vi "CMD_Codec.vi"() -> ()   [LabVIEW 2025]
uses:
  <vilib>/addons/JSON API/JSON Value/Set from JSON string.vi
  <vilib>/addons/JSON API/JSON Value/JSON Value.lvclass
  <vilib>/addons/JSON API/JSON Value/Get sub-Item by names.vi
  <vilib>/addons/JSON API/JSON Scalar/Get as Text.vi
  <vilib>/addons/JSON API/Get Polymorphic/JSON GetSet.lvlib
  <vilib>/addons/JSON API/JSON Scalar/JSON Scalar.lvclass
  <vilib>/addons/JSON API/JSON Scalar/Set String.vi
panel:
  out "CMD":string
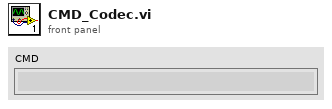
[diagram p1: front panel]
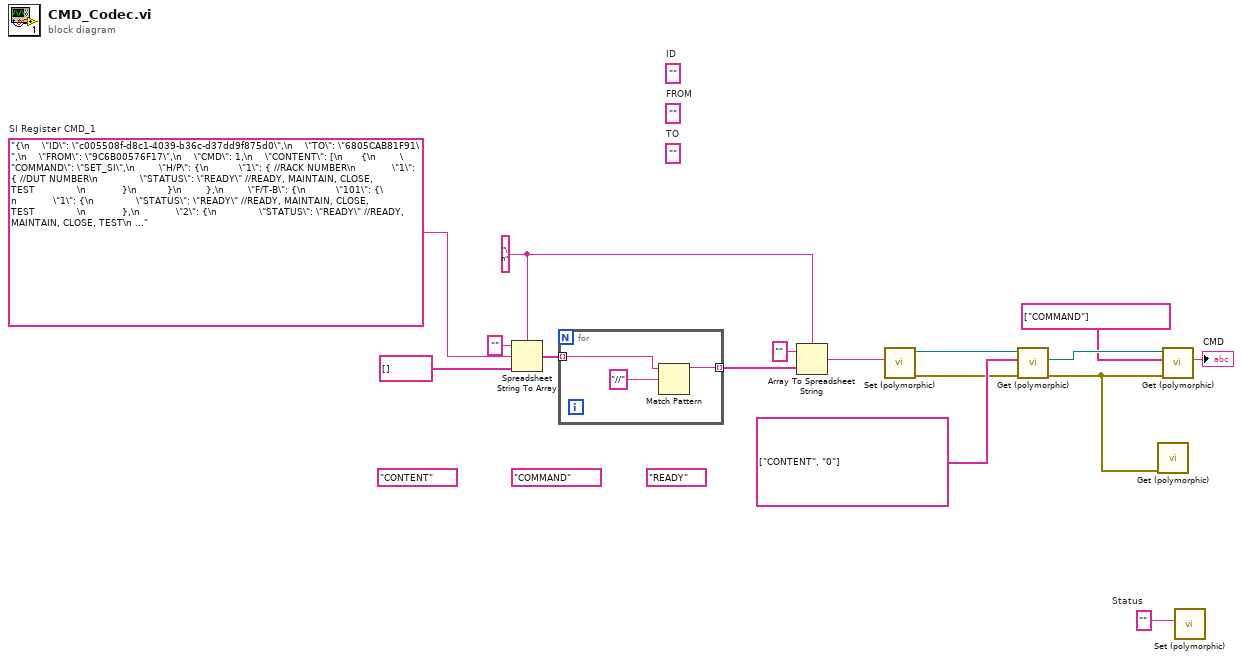
[diagram p0: block diagram]
diagram:
  (unwired) "COMMAND" ("Combo Box")
  (unwired) "READY" ("Combo Box")
  (unwired) "CONTENT" ("Combo Box")
  w1 = ""  # Status
  (unwired) ""  # TO
  (unwired) ""  # FROM
  (unwired) ""  # ID
  w11 = "\n" ("delimiter (Tab)")
  w15 = "{\n    \"ID\": \"c005508f-d8c1-4039-b36c-d37dd9f875d0\",\n    \"TO\": \"6805CAB81F91\",\n    \"FROM\": \"9C6B00576F17\",\n    \"CMD\": 1,\n    \"CONTENT\": [\n      {\n        \"COMMAND\": \"SET_SI\",\n        \"H/P\": {\n          \"1\": { //RACK NUMBER\n            \"1\": { //DUT NUMBER\n              \"STATUS\": \"READY\" //READY, MAINTAIN, CLOSE, TEST              \n            }\n          }\n        },\n        \"F/T-B\": {\n          \"101\": {\n            \"1\": {\n              \"STATUS\": \"READY\" //READY, MAINTAIN, CLOSE, TEST              \n            },\n            \"2\": {\n              \"STATUS\": \"READY\" //READY, MAINTAIN, CLOSE, TEST\n            },\n            \"3\": {\n              \"STATUS\": \"READY\" //READY, MAINTAIN, CLOSE, TEST\n            },\n            \"4\": {\n              \"STATUS\": \"READY\" //READY, MAINTAIN, CLOSE, TEST\n            },\n            \"5\": {\n              \"STATUS\": \"READY\" //READY, MAINTAIN, CLOSE, TEST\n            }\n          },\n          \"102\": {\n            \"1\": {\n              \"STATUS\": \"READY\" //READY, MAINTAIN, CLOSE, TEST              \n            },\n            \"2\": {\n              \"STATUS\": \"READY\" //READY, MAINTAIN, CLOSE, TEST\n            },\n            \"3\": {\n              \"STATUS\": \"READY\" //READY, MAINTAIN, CLOSE, TEST\n            },\n            \"4\": {\n              \"STATUS\": \"READY\" //READY, MAINTAIN, CLOSE, TEST\n            },\n            \"5\": {\n              \"STATUS\": \"READY\" //READY, MAINTAIN, CLOSE, TEST\n            }\n          },\n          \"103\": {\n            \"1\": {\n              \"STATUS\": \"READY\" //READY, MAINTAIN, CLOSE, TEST              \n            },\n            \"2\": {\n              \"STATUS\": \"READY\" //READY, MAINTAIN, CLOSE, TEST\n            },\n            \"3\": {\n              \"STATUS\": \"READY\" //READY, MAINTAIN, CLOSE, TEST\n            },\n            \"4\": {\n              \"STATUS\": \"READY\" //READY, MAINTAIN, CLOSE, TEST\n            },\n            \"5\": {\n              \"STATUS\": \"READY\" //READY, MAINTAIN, CLOSE, TEST\n            }\n          },\n          \"104\": {\n            \"1\": {\n              \"STATUS\": \"READY\" //READY, MAINTAIN, CLOSE, TEST              \n            },\n            \"2\": {\n              \"STATUS\": \"READY\" //READY, MAINTAIN, CLOSE, TEST\n            },\n            \"3\": {\n              \"STATUS\": \"READY\" //READY, MAINTAIN, CLOSE, TEST\n            },\n            \"4\": {\n              \"STATUS\": \"READY\" //READY, MAINTAIN, CLOSE, TEST\n            },\n            \"5\": {\n              \"STATUS\": \"READY\" //READY, MAINTAIN, CLOSE, TEST\n            }\n          },\n          \"105\": {\n            \"1\": {\n              \"STATUS\": \"READY\" //READY, MAINTAIN, CLOSE, TEST              \n            },\n            \"2\": {\n              \"STATUS\": \"READY\" //READY, MAINTAIN, CLOSE, TEST\n            },\n            \"3\": {\n              \"STATUS\": \"READY\" //READY, MAINTAIN, CLOSE, TEST\n            },\n            \"4\": {\n              \"STATUS\": \"READY\" //READY, MAINTAIN, CLOSE, TEST\n            },\n            \"5\": {\n              \"STATUS\": \"READY\" //READY, MAINTAIN, CLOSE, TEST\n            }\n          },\n          \"106\": {\n            \"1\": {\n              \"STATUS\": \"READY\" //READY, MAINTAIN, CLOSE, TEST              \n            },\n            \"2\": {\n              \"STATUS\": \"READY\" //READY, MAINTAIN, CLOSE, TEST\n            },\n            \"3\": {\n              \"STATUS\": \"READY\" //READY, MAINTAIN, CLOSE, TEST\n            },\n            \"4\": {\n              \"STATUS\": \"READY\" //READY, MAINTAIN, CLOSE, TEST\n            },\n            \"5\": {\n              \"STATUS\": \"READY\" //READY, MAINTAIN, CLOSE, TEST\n            }\n          },\n          \"107\": {\n            \"1\": {\n              \"STATUS\": \"READY\" //READY, MAINTAIN, CLOSE, TEST              \n            },\n            \"2\": {\n              \"STATUS\": \"READY\" //READY, MAINTAIN, CLOSE, TEST\n            },\n            \"3\": {\n              \"STATUS\": \"READY\" //READY, MAINTAIN, CLOSE, TEST\n            },\n            \"4\": {\n              \"STATUS\": \"READY\" //READY, MAINTAIN, CLOSE, TEST\n            },\n            \"5\": {\n              \"STATUS\": \"READY\" //READY, MAINTAIN, CLOSE, TEST\n            }\n          },\n          \"108\": {\n            \"1\": {\n              \"STATUS\": \"READY\" //READY, MAINTAIN, CLOSE, TEST              \n            },\n            \"2\": {\n              \"STATUS\": \"READY\" //READY, MAINTAIN, CLOSE, TEST\n            },\n            \"3\": {\n              \"STATUS\": \"READY\" //READY, MAINTAIN, CLOSE, TEST\n            },\n            \"4\": {\n              \"STATUS\": \"READY\" //READY, MAINTAIN, CLOSE, TEST\n            },\n            \"5\": {\n              \"STATUS\": \"READY\" //READY, MAINTAIN, CLOSE, TEST\n            }\n          },\n          \"109\": {\n            \"1\": {\n              \"STATUS\": \"READY\" //READY, MAINTAIN, CLOSE, TEST              \n            },\n            \"2\": {\n              \"STATUS\": \"READY\" //READY, MAINTAIN, CLOSE, TEST\n            },\n            \"3\": {\n              \"STATUS\": \"READY\" //READY, MAINTAIN, CLOSE, TEST\n            },\n            \"4\": {\n              \"STATUS\": \"READY\" //READY, MAINTAIN, CLOSE, TEST\n            },\n            \"5\": {\n              \"STATUS\": \"READY\" //READY, MAINTAIN, CLOSE, TEST\n            }\n          },\n          \"110\": {\n            \"1\": {\n              \"STATUS\": \"READY\" //READY, MAINTAIN, CLOSE, TEST              \n            },\n            \"2\": {\n              \"STATUS\": \"READY\" //READY, MAINTAIN, CLOSE, TEST\n            },\n            \"3\": {\n              \"STATUS\": \"READY\" //READY, MAINTAIN, CLOSE, TEST\n            },\n            \"4\": {\n              \"STATUS\": \"READY\" //READY, MAINTAIN, CLOSE, TEST\n            },\n            \"5\": {\n              \"STATUS\": \"READY\" //READY, MAINTAIN, CLOSE, TEST\n            }\n          },\n          \"111\": {\n            \"1\": {\n              \"STATUS\": \"READY\" //READY, MAINTAIN, CLOSE, TEST              \n            },\n            \"2\": {\n              \"STATUS\": \"READY\" //READY, MAINTAIN, CLOSE, TEST\n            },\n            \"3\": {\n              \"STATUS\": \"READY\" //READY, MAINTAIN, CLOSE, TEST\n            },\n            \"4\": {\n              \"STATUS\": \"READY\" //READY, MAINTAIN, CLOSE, TEST\n            },\n            \"5\": {\n              \"STATUS\": \"READY\" //READY, MAINTAIN, CLOSE, TEST\n            }\n          },\n          \"112\": {\n            \"1\": {\n              \"STATUS\": \"READY\" //READY, MAINTAIN, CLOSE, TEST              \n            },\n            \"2\": {\n              \"STATUS\": \"READY\" //READY, MAINTAIN, CLOSE, TEST\n            },\n            \"3\": {\n              \"STATUS\": \"READY\" //READY, MAINTAIN, CLOSE, TEST\n            },\n            \"4\": {\n              \"STATUS\": \"READY\" //READY, MAINTAIN, CLOSE, TEST\n            },\n            \"5\": {\n              \"STATUS\": \"READY\" //READY, MAINTAIN, CLOSE, TEST\n            }\n          }\n        },\n        \"F/T\": {\n          \"201\": {\n            \"1\": {\n              \"STATUS\": \"READY\" //READY, MAINTAIN, CLOSE, TEST              \n            },\n            \"2\": {\n              \"STATUS\": \"READY\" //READY, MAINTAIN, CLOSE, TEST\n            },\n            \"3\": {\n              \"STATUS\": \"READY\" //READY, MAINTAIN, CLOSE, TEST\n            },\n            \"4\": {\n              \"STATUS\": \"READY\" //READY, MAINTAIN, CLOSE, TEST\n            },\n            \"5\": {\n              \"STATUS\": \"READY\" //READY, MAINTAIN, CLOSE, TEST\n            }\n          },\n          \"202\": {\n            \"1\": {\n              \"STATUS\": \"READY\" //READY, MAINTAIN, CLOSE, TEST              \n            },\n            \"2\": {\n              \"STATUS\": \"READY\" //READY, MAINTAIN, CLOSE, TEST\n            },\n            \"3\": {\n              \"STATUS\": \"READY\" //READY, MAINTAIN, CLOSE, TEST\n            },\n            \"4\": {\n              \"STATUS\": \"READY\" //READY, MAINTAIN, CLOSE, TEST\n            },\n            \"5\": {\n              \"STATUS\": \"READY\" //READY, MAINTAIN, CLOSE, TEST\n            }\n          },\n          \"203\": {\n            \"1\": {\n              \"STATUS\": \"READY\" //READY, MAINTAIN, CLOSE, TEST              \n            },\n            \"2\": {\n              \"STATUS\": \"READY\" //READY, MAINTAIN, CLOSE, TEST\n            },\n            \"3\": {\n              \"STATUS\": \"READY\" //READY, MAINTAIN, CLOSE, TEST\n            },\n            \"4\": {\n              \"STATUS\": \"READY\" //READY, MAINTAIN, CLOSE, TEST\n            },\n            \"5\": {\n              \"STATUS\": \"READY\" //READY, MAINTAIN, CLOSE, TEST\n            }\n          },\n          \"204\": {\n            \"1\": {\n              \"STATUS\": \"READY\" //READY, MAINTAIN, CLOSE, TEST              \n            },\n            \"2\": {\n              \"STATUS\": \"READY\" //READY, MAINTAIN, CLOSE, TEST\n            },\n            \"3\": {\n              \"STATUS\": \"READY\" //READY, MAINTAIN, CLOSE, TEST\n            },\n            \"4\": {\n              \"STATUS\": \"READY\" //READY, MAINTAIN, CLOSE, TEST\n            },\n            \"5\": {\n              \"STATUS\": \"READY\" //READY, MAINTAIN, CLOSE, TEST\n            }\n          },\n          \"205\": {\n            \"1\": {\n              \"STATUS\": \"READY\" //READY, MAINTAIN, CLOSE, TEST              \n            },\n            \"2\": {\n              \"STATUS\": \"READY\" //READY, MAINTAIN, CLOSE, TEST\n            },\n            \"3\": {\n              \"STATUS\": \"READY\" //READY, MAINTAIN, CLOSE, TEST\n            },\n            \"4\": {\n              \"STATUS\": \"READY\" //READY, MAINTAIN, CLOSE, TEST\n            },\n            \"5\": {\n              \"STATUS\": \"READY\" //READY, MAINTAIN, CLOSE, TEST\n            }\n          },\n          \"206\": {\n            \"1\": {\n              \"STATUS\": \"READY\" //READY, MAINTAIN, CLOSE, TEST              \n            },\n            \"2\": {\n              \"STATUS\": \"READY\" //READY, MAINTAIN, CLOSE, TEST\n            },\n            \"3\": {\n              \"STATUS\": \"READY\" //READY, MAINTAIN, CLOSE, TEST\n            },\n            \"4\": {\n              \"STATUS\": \"READY\" //READY, MAINTAIN, CLOSE, TEST\n            },\n            \"5\": {\n              \"STATUS\": \"READY\" //READY, MAINTAIN, CLOSE, TEST\n            }\n          },\n          \"207\": {\n            \"1\": {\n              \"STATUS\": \"READY\" //READY, MAINTAIN, CLOSE, TEST              \n            },\n            \"2\": {\n              \"STATUS\": \"READY\" //READY, MAINTAIN, CLOSE, TEST\n            },\n            \"3\": {\n              \"STATUS\": \"READY\" //READY, MAINTAIN, CLOSE, TEST\n            },\n            \"4\": {\n              \"STATUS\": \"READY\" //READY, MAINTAIN, CLOSE, TEST\n            },\n            \"5\": {\n              \"STATUS\": \"READY\" //READY, MAINTAIN, CLOSE, TEST\n            }\n          },\n          \"208\": {\n            \"1\": {\n              \"STATUS\": \"READY\" //READY, MAINTAIN, CLOSE, TEST              \n            },\n            \"2\": {\n              \"STATUS\": \"READY\" //READY, MAINTAIN, CLOSE, TEST\n            },\n            \"3\": {\n              \"STATUS\": \"READY\" //READY, MAINTAIN, CLOSE, TEST\n            },\n            \"4\": {\n              \"STATUS\": \"READY\" //READY, MAINTAIN, CLOSE, TEST\n            },\n            \"5\": {\n              \"STATUS\": \"READY\" //READY, MAINTAIN, CLOSE, TEST\n            }\n          },\n          \"209\": {\n            \"1\": {\n              \"STATUS\": \"READY\" //READY, MAINTAIN, CLOSE, TEST              \n            },\n            \"2\": {\n              \"STATUS\": \"READY\" //READY, MAINTAIN, CLOSE, TEST\n            },\n            \"3\": {\n              \"STATUS\": \"READY\" //READY, MAINTAIN, CLOSE, TEST\n            },\n            \"4\": {\n              \"STATUS\": \"READY\" //READY, MAINTAIN, CLOSE, TEST\n            },\n            \"5\": {\n              \"STATUS\": \"READY\" //READY, MAINTAIN, CLOSE, TEST\n            }\n          },\n          \"210\": {\n            \"1\": {\n              \"STATUS\": \"READY\" //READY, MAINTAIN, CLOSE, TEST              \n            },\n            \"2\": {\n              \"STATUS\": \"READY\" //READY, MAINTAIN, CLOSE, TEST\n            },\n            \"3\": {\n              \"STATUS\": \"READY\" //READY, MAINTAIN, CLOSE, TEST\n            },\n            \"4\": {\n              \"STATUS\": \"READY\" //READY, MAINTAIN, CLOSE, TEST\n            },\n            \"5\": {\n              \"STATUS\": \"READY\" //READY, MAINTAIN, CLOSE, TEST\n            }\n          },\n          \"211\": {\n            \"1\": {\n              \"STATUS\": \"READY\" //READY, MAINTAIN, CLOSE, TEST              \n            },\n            \"2\": {\n              \"STATUS\": \"READY\" //READY, MAINTAIN, CLOSE, TEST\n            },\n            \"3\": {\n              \"STATUS\": \"READY\" //READY, MAINTAIN, CLOSE, TEST\n            },\n            \"4\": {\n              \"STATUS\": \"READY\" //READY, MAINTAIN, CLOSE, TEST\n            },\n            \"5\": {\n              \"STATUS\": \"READY\" //READY, MAINTAIN, CLOSE, TEST\n            }\n          },\n          \"212\": {\n            \"1\": {\n              \"STATUS\": \"READY\" //READY, MAINTAIN, CLOSE, TEST              \n            },\n            \"2\": {\n              \"STATUS\": \"READY\" //READY, MAINTAIN, CLOSE, TEST\n            },\n            \"3\": {\n              \"STATUS\": \"READY\" //READY, MAINTAIN, CLOSE, TEST\n            },\n            \"4\": {\n              \"STATUS\": \"READY\" //READY, MAINTAIN, CLOSE, TEST\n            },\n            \"5\": {\n              \"STATUS\": \"READY\" //READY, MAINTAIN, CLOSE, TEST\n            }\n          }\n        }\n      }\n    ],\n    \"STATUS\": \"\",\n    \"ERRCODE\": \"\",\n    \"ERRMSG\": \"\",\n    \"TIMESTAMP\": \"1758590005\"\n  }"  # SI Register CMD_1
  n1 = Spreadsheet String To Array(delimiter (Tab)=w11, format string="", spreadsheet string=w15, array type (2D Dbl)=string[] []) -> (array=w13:string[])
  n2 = for {
    tunnel: w13 -> [w19] mode=indexing
    tunnel: [w17] -> w12 mode=indexing
    n3 = Match Pattern(string=w19, regular expression="//") -> (before substring=w17:string)  [unwired: 1 in, 3 out]
  }
  n4 = Array To Spreadsheet String(delimiter (Tab)=w11, array=w12, 3:"" ("format string")) -> (spreadsheet string=w9:string)
  n5 = call-poly <vilib>:"Set (polymorphic).vi"("JSON stream"=w9) -> ("error out"=w3:errorcluster, "JSON Value out"=w8:refnum<class "JSON Value.lvclass">)  [unwired: 8 in, 1 out]
  n6 = call-poly <vilib>:"Get (polymorphic).vi"("error in (no error)"=w3, "Name Array"=string[] ["CONTENT", "0"], "JSON Value In"=w8) -> ("error out"=w2:errorcluster, "Value"=w6:refnum<class "JSON Value.lvclass">)  [unwired: 5 in, 2 out]
  n7 = call-poly <vilib>:"Get (polymorphic).vi"("error in (no error)"=w2) -> ()  [unwired: 8 in, 3 out]
  n8 = call-poly <vilib>:"Get (polymorphic).vi"("error in (no error)"=w2, "Name Array"=string[] ["COMMAND"], "JSON Scalar in"=w6) -> ("LabVIEW Text"=→"CMD":string)  [unwired: 6 in, 2 out]
  n9 = call-poly <vilib>:"Set (polymorphic).vi"("String"=w1) -> ()  [unwired: 9 in, 2 out]
